vi "Set adquisicion Config.vi"(8 "error in (no error)":errorcluster, 10 "config":T1={"sampling info"={"Fs"=1000.0, "#s"=1000.0}, "signal type"=enum."Sine Wave", "square wave duty cycle (%)"=50.0, "offset"=0.0, "frequency"=10.0, "amplitude"=1.0, "phase"=0.0}) -> (0 "error out":errorcluster)   [LabVIEW 2019]
doc: "sets teh waveform\n_____\nCreated using Delacor QMH Event Scripter 5.0.0.112."
uses:
  Set adquisicion Config Argument--cluster.ctl
  Adquisiion2.lvlib
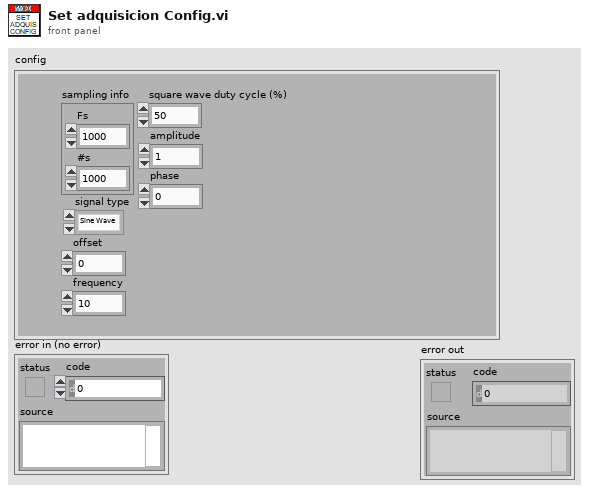
[diagram p1: front panel]
types:
  T1 = cluster{"sampling info":cluster{"Fs":dbl, "#s":dbl}, "signal type":enum16{"Sine Wave", "Triangle Wave", "Square Wave", "Sawtooth Wave"}, "square wave duty cycle (%)":dbl, "offset":dbl, "frequency":dbl, "amplitude":dbl, "phase":dbl}
  T2 = typedef "Set adquisicion Config Argument--cluster.ctl" = cluster{"config":cluster{"sampling info":cluster{"Fs":dbl, "#s":dbl}, "signal type":enum16{"Sine Wave", "Triangle Wave", "Square Wave", "Sawtooth Wave"}, "square wave duty cycle (%)":dbl, "offset":dbl, "frequency":dbl, "amplitude":dbl, "phase":dbl}}
  T3 = typedef "Adquisiion2.lvlib/Request Events--cluster.ctl" = cluster{"Stop Module":refnum<user-event>, "Show Panel":refnum<user-event>, "Hide Panel":refnum<user-event>, "Get Module Execution Status":refnum<user-event>, "Show Diagram":refnum<user-event>, "Start helper loop":refnum<user-event>, "stop helper loop":refnum<user-event>}
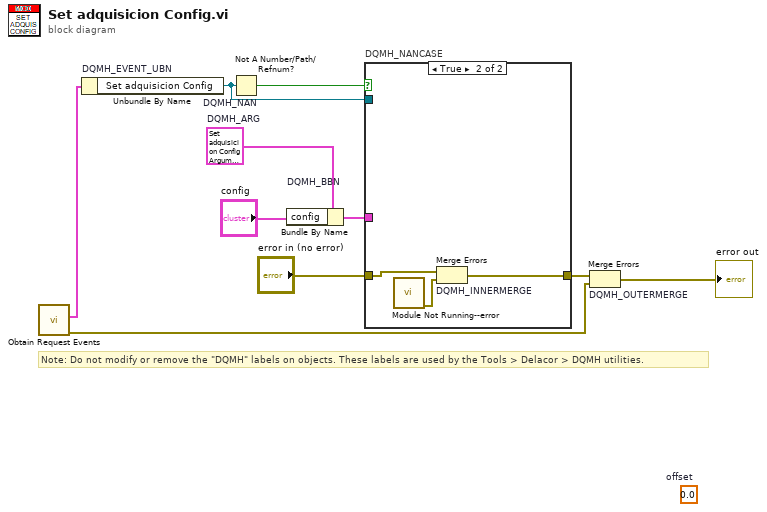
[diagram p0: block diagram]
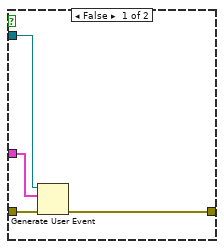
[diagram p2: hidden frame]
diagram:
  (unwired) 0.0  # offset
  w4 = T2 {"config"={"sampling info"={"Fs"=1000.0, "#s"=1000.0}, "signal type"=enum."Sine Wave", "square wave duty cycle (%)"=50.0, "offset"=0.0, "frequency"=10.0, "amplitude"=1.0, "phase"=0.0}}  # DQMH_ARG
  # "Note: Do not modify or remove the \"DQMH\" labels on objects. These labels are used by the Tools > Delacor > DQMH utilities."
  n1 = call "Obtain Request Events.vi"() -> ("error out"=w3:errorcluster, "Adquisiion2 Request Events"=w2:T3)  [unwired: 10 in]
  n2 = Unbundle By Name "DQMH_EVENT_UBN"(w2) -> ("Set adquisicion Config"=w6:refnum<user-event>)
  n3 = Not A Number/Path/Refnum? "DQMH_NAN"(number/path/refnum=w6) -> (NaN/Path/Refnum?=w7:bool)
  n4 = Bundle By Name "DQMH_BBN"(cluster=w4, "config"="config") -> (w8:T2)
  n5 = case "DQMH_NANCASE" shown="True" w7 {
    tunnel: "error in (no error)" -> [w14 w17]
    tunnel: [w13 w16] -> w5
    tunnel: w6 -> [w12 _]
    tunnel: w8 -> [w11 _]
    frame False {
      n6 = Generate User Event(user event=w12, event data cluster=w11, error in=w14) -> (error out=w13:errorcluster)  [unwired: 1 in, 1 out]
    }
    frame True {
      n7 = call "Module Not Running--error.vi"() -> ("error out"=w15:errorcluster)  [unwired: 11 in]
      n8 = Merge Errors "DQMH_INNERMERGE"(w17, w15) -> (w16:errorcluster)
    }
  }
  n9 = Merge Errors "DQMH_OUTERMERGE"(w5, w3) -> (→"error out":errorcluster)
